vi "Rising Edge Latch.vi"(10 "S Rising Edge":bool[](array[boolean])=[FALSE, FALSE, FALSE, FALSE], 11 "Reset":bool) -> (2 "Rising Edge Out":bool[](array[boolean]))   [LabVIEW 2012]
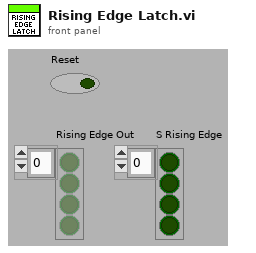
[diagram p1: front panel]
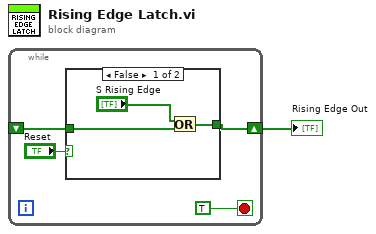
[diagram p0: block diagram]
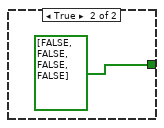
[diagram p2: hidden frame]
diagram:
  n1 = while {
    shift-right: [w3] -> w1
    shift-left: _ -> [w4]
    stop <- TRUE stop-if-true
    n2 = case shown="False" "Reset" {
      tunnel: w4 -> [w8 _]
      tunnel: [w7 bool[] [FALSE, FALSE, FALSE, FALSE] ("Rising Edge")] -> w3
      frame False {
        n3 = Or(x="S Rising Edge", y=w8) -> (x .or. y?=w7:bool[])
      }
      frame True {
      }
    }
  }
  "Rising Edge Out" <- w1
